vi "Pow Meas Close.vi"(0 "task/channels in":refnum<k21>, 11 "error in (no error)":errorcluster) -> (15 "error out":errorcluster)   [LabVIEW 2021, in "Power Measurement_Z Power Module.lvlib"]
uses:
  Power Measurement_Z Power Module.lvlib
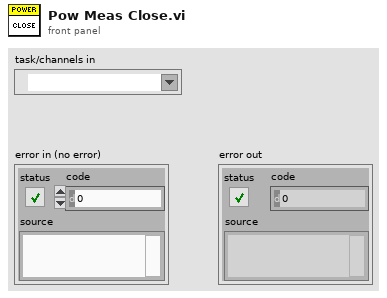
[diagram p1: front panel]
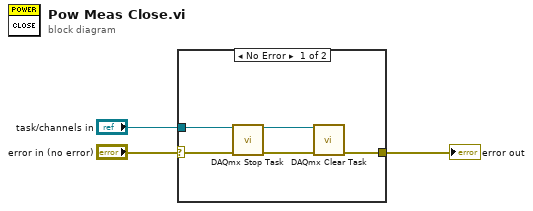
[diagram p0: block diagram]
diagram:
  n1 = case shown="No Error" "error in (no error)" {
    selector: "error in (no error)" -> [w8 w9]
    tunnel: "task/channels in" -> [w5 _]
    tunnel: [w4 w9] -> w1
    frame No Error {
      n2 = call <vilib>:"DAQmx Stop Task.vi"("task/channels in"=w5, "error in"=w8) -> ("task out"=w6:refnum<k21>, "error out"=w7:errorcluster)  [unwired: 12 in]
      n3 = call <vilib>:"DAQmx Clear Task.vi"("task in"=w6, "error in"=w7) -> ("error out"=w4:errorcluster)  [unwired: 13 in]
    }
    frame Error {
    }
  }
  "error out" <- w1
